vi "Create_TreeNode_PN.vi"(1 "Input cluster":T1) -> (0 "TreeNode out":T2)   [LabVIEW 2011]
uses:
  TreeNode2D.ctl
  TreeNode2D Input Cluster.ctl
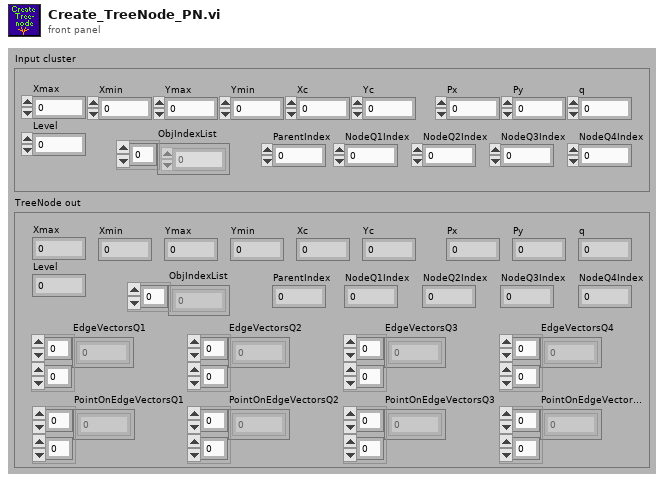
[diagram p1: front panel]
types:
  T1 = typedef "TreeNode2D Input Cluster.ctl" = cluster{"Xmax":dbl, "Xmin":dbl, "Ymax":dbl, "Ymin":dbl, "Xc":dbl, "Yc":dbl, "Px":dbl, "Py":dbl, "q":dbl, "Level":i32, "ObjIndexList":i32[], "ParentIndex":i32, "NodeQ1Index":i32, "NodeQ2Index":i32, "NodeQ3Index":i32, "NodeQ4Index":i32}
  T2 = typedef "TreeNode2D.ctl" = cluster{"Xmax":dbl, "Xmin":dbl, "Ymax":dbl, "Ymin":dbl, "Xc":dbl, "Yc":dbl, "Px":dbl, "Py":dbl, "q":dbl, "Level":i32, "ObjIndexList":i32[], "ParentIndex":i32, "NodeQ1Index":i32, "NodeQ2Index":i32, "NodeQ3Index":i32, "NodeQ4Index":i32, "EdgeVectorsQ1":dbl[][], "EdgeVectorsQ2":dbl[][], "EdgeVectorsQ3":dbl[][], "EdgeVectorsQ4":dbl[][], "PointOnEdgeVectorsQ1":dbl[][], "PointOnEdgeVectorsQ2":dbl[][], "PointOnEdgeVectorsQ3":dbl[][], "PointOnEdgeVectorsQ4":dbl[][]}
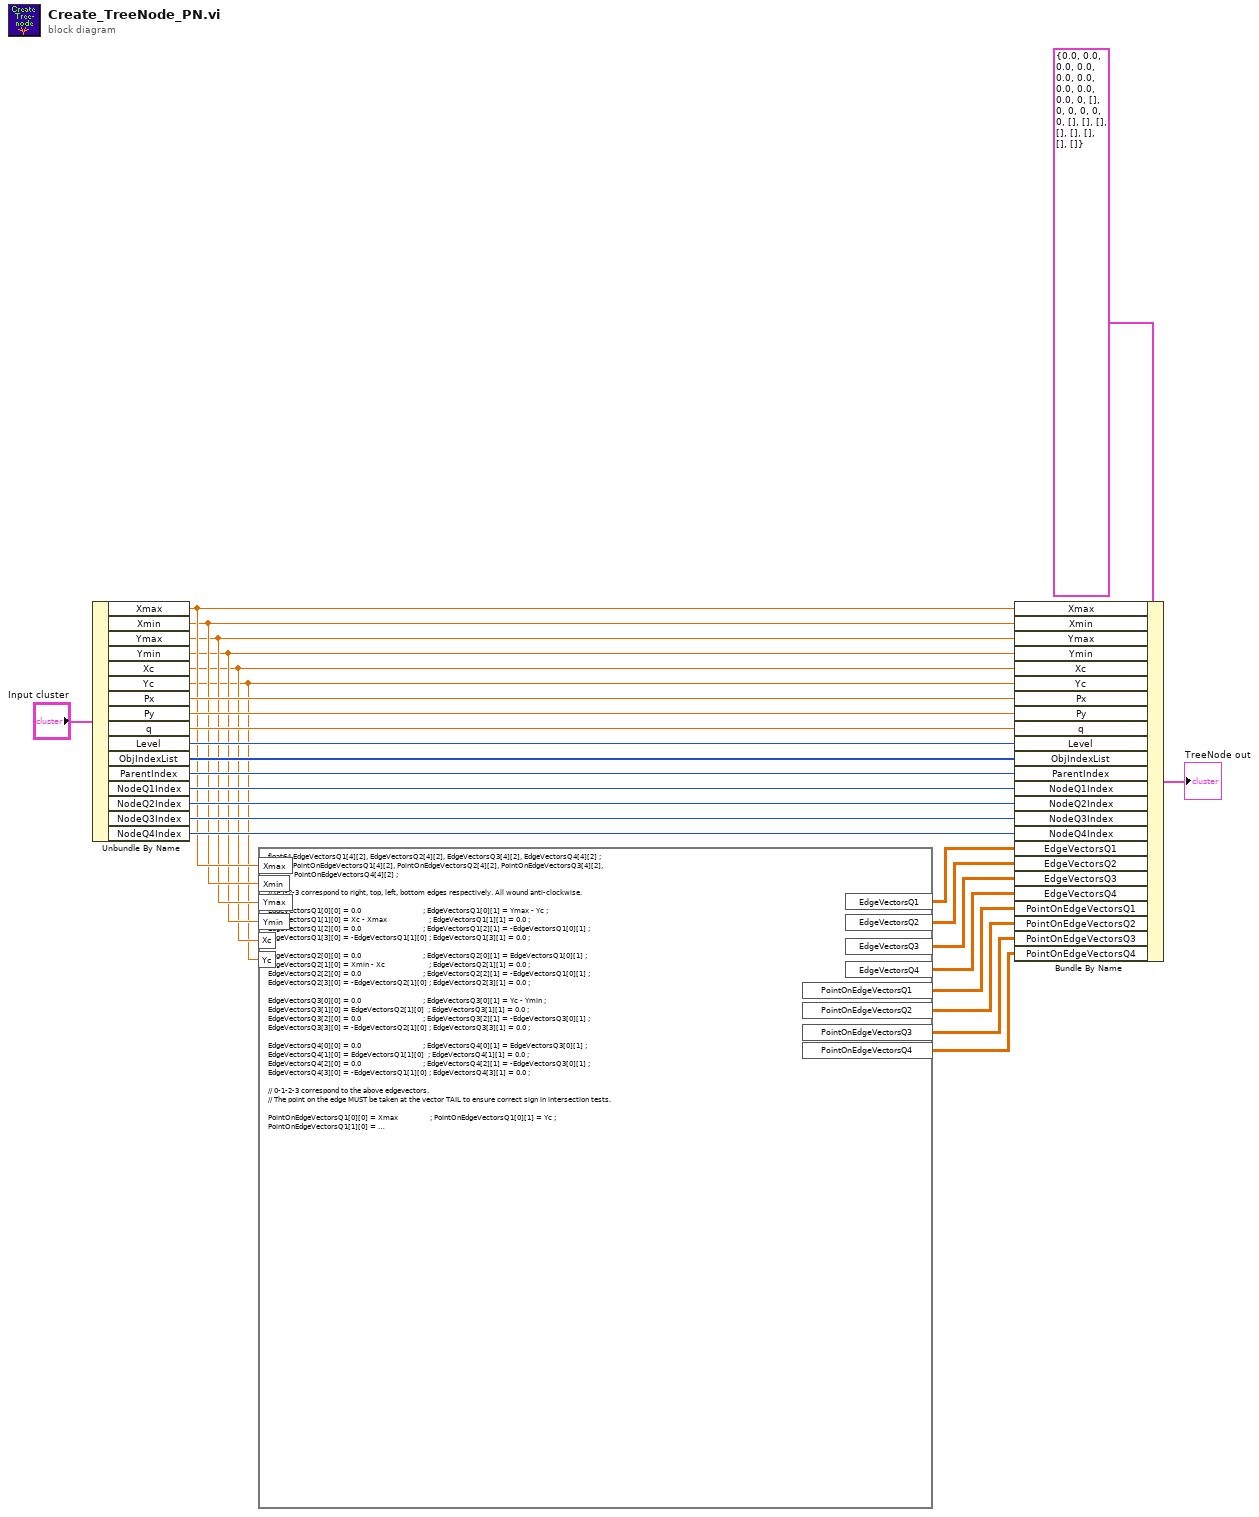
[diagram p0: block diagram]
diagram:
  n1 = Unbundle By Name("Input cluster") -> ("Xmax"=w13:dbl, "Xmin"=w12:dbl, "Ymax"=w11:dbl, "Ymin"=w10:dbl, "Xc"=w9:dbl, "Yc"=w8:dbl, "Px"=w24:dbl, "Py"=w23:dbl, "q"=w22:dbl, "Level"=w21:i32, "ObjIndexList"=w20:i32[], "ParentIndex"=w19:i32, "NodeQ1Index"=w18:i32, "NodeQ2Index"=w17:i32, "NodeQ3Index"=w16:i32, "NodeQ4Index"=w15:i32)
  n2 = formula code="float64 EdgeVectorsQ1[4][2], EdgeVectorsQ2[4][2], EdgeVectorsQ3[4][2], EdgeVectorsQ4[4][2] ;\nfloat64 PointOnEdgeVectorsQ1[4][2], PointOnEdgeVectorsQ2[4][2], PointOnEdgeVectorsQ3[4][2], \n             PointOnEdgeVectorsQ4[4][2] ;\n\n// 0-1-2-3 correspond to right, top, left, bottom edges respectively. All wound anti-clockwise.\n\nEdgeVectorsQ1[0][0] = 0.0                               ; EdgeVectorsQ1[0][1] = Ymax - Yc ;\nEdgeVectorsQ1[1][0] = Xc - Xmax                     ; EdgeVectorsQ1[1][1] = 0.0 ;\nEdgeVectorsQ1[2][0] = 0.0                               ; EdgeVectorsQ1[2][1] = -EdgeVectorsQ1[0][1] ;\nEdgeVectorsQ1[3][0] = -EdgeVectorsQ1[1][0] ; EdgeVectorsQ1[3][1] = 0.0 ;\n\nEdgeVectorsQ2[0][0] = 0.0                               ; EdgeVectorsQ2[0][1] = EdgeVectorsQ1[0][1] ;\nEdgeVectorsQ2[1][0] = Xmin - Xc                      ; EdgeVectorsQ2[1][1] = 0.0 ;\nEdgeVectorsQ2[2][0] = 0.0                               ; EdgeVectorsQ2[2][1] = -EdgeVectorsQ1[0][1] ;\nEdgeVectorsQ2[3][0] = -EdgeVectorsQ2[1][0] ; EdgeVectorsQ2[3][1] = 0.0 ;\n\nEdgeVectorsQ3[0][0] = 0.0                               ; EdgeVectorsQ3[0][1] = Yc - Ymin ;\nEdgeVectorsQ3[1][0] = EdgeVectorsQ2[1][0]  ; EdgeVectorsQ3[1][1] = 0.0 ;\nEdgeVectorsQ3[2][0] = 0.0                               ; EdgeVectorsQ3[2][1] = -EdgeVectorsQ3[0][1] ;\nEdgeVectorsQ3[3][0] = -EdgeVectorsQ2[1][0] ; EdgeVectorsQ3[3][1] = 0.0 ;\n\nEdgeVectorsQ4[0][0] = 0.0                               ; EdgeVectorsQ4[0][1] = EdgeVectorsQ3[0][1] ;\nEdgeVectorsQ4[1][0] = EdgeVectorsQ1[1][0]  ; EdgeVectorsQ4[1][1] = 0.0 ;\nEdgeVectorsQ4[2][0] = 0.0                               ; EdgeVectorsQ4[2][1] = -EdgeVectorsQ3[0][1] ;\nEdgeVectorsQ4[3][0] = -EdgeVectorsQ1[1][0] ; EdgeVectorsQ4[3][1] = 0.0 ;\n\n// 0-1-2-3 correspond to the above edgevectors.\n// The point on the edge MUST be taken at the vector TAIL to ensure correct sign in intersection tests.\n\nPointOnEdgeVectorsQ1[0][0] = Xmax                ; PointOnEdgeVectorsQ1[0][1] = Yc ;\nPointOnEdgeVectorsQ1[1][0] = Xmax                ; PointOnEdgeVectorsQ1[1][1] = Ymax ;\nPointOnEdgeVectorsQ1[2][0] = Xc                     ; PointOnEdgeVectorsQ1[2][1] = Ymax ;\nPointOnEdgeVectorsQ1[3][0] = Xc                     ; PointOnEdgeVectorsQ1[3][1] = Yc ;\n\nPointOnEdgeVectorsQ2[0][0] = Xc                     ; PointOnEdgeVectorsQ2[0][1] = Yc ;\nPointOnEdgeVectorsQ2[1][0] = Xc                     ; PointOnEdgeVectorsQ2[1][1] = Ymax ;\nPointOnEdgeVectorsQ2[2][0] = Xmin                 ; PointOnEdgeVectorsQ2[2][1] = Ymax ;\nPointOnEdgeVectorsQ2[3][0] = Xmin                 ; PointOnEdgeVectorsQ2[3][1] = Yc ;\n\nPointOnEdgeVectorsQ3[0][0] = Xc                     ; PointOnEdgeVectorsQ3[0][1] = Ymin ;\nPointOnEdgeVectorsQ3[1][0] = Xc                     ; PointOnEdgeVectorsQ3[1][1] = Yc ;\nPointOnEdgeVectorsQ3[2][0] = Xmin                 ; PointOnEdgeVectorsQ3[2][1] = Yc ;\nPointOnEdgeVectorsQ3[3][0] = Xmin                 ; PointOnEdgeVectorsQ3[3][1] = Ymin ;\n\nPointOnEdgeVectorsQ4[0][0] = Xmax                ; PointOnEdgeVectorsQ4[0][1] = Ymin ;\nPointOnEdgeVectorsQ4[1][0] = Xmax                ; PointOnEdgeVectorsQ4[1][1] = Yc ;\nPointOnEdgeVectorsQ4[2][0] = Xc                     ; PointOnEdgeVectorsQ4[2][1] = Yc ;\nPointOnEdgeVectorsQ4[3][0] = Xc                     ; PointOnEdgeVectorsQ4[3][1] = Ymin ;"("Xmax"=w13, "Xmin"=w12, "Ymax"=w11, "Ymin"=w10, "Xc"=w9, "Yc"=w8) -> ("EdgeVectorsQ1"=w14:dbl[][], "EdgeVectorsQ2"=w7:dbl[][], "EdgeVectorsQ3"=w6:dbl[][], "EdgeVectorsQ4"=w5:dbl[][], "PointOnEdgeVectorsQ1"=w4:dbl[][], "PointOnEdgeVectorsQ2"=w3:dbl[][], "PointOnEdgeVectorsQ3"=w2:dbl[][], "PointOnEdgeVectorsQ4"=w1:dbl[][])
  n3 = Bundle By Name(cluster=T2 {"Xmax"=0.0, "Xmin"=0.0, "Ymax"=0.0, "Ymin"=0.0, "Xc"=0.0, "Yc"=0.0, "Px"=0.0, "Py"=0.0, "q"=0.0, "Level"=0, "ObjIndexList"=[], "ParentIndex"=0, "NodeQ1Index"=0, "NodeQ2Index"=0, "NodeQ3Index"=0, "NodeQ4Index"=0, "EdgeVectorsQ1"=[], "EdgeVectorsQ2"=[], "EdgeVectorsQ3"=[], "EdgeVectorsQ4"=[], "PointOnEdgeVectorsQ1"=[], "PointOnEdgeVectorsQ2"=[], "PointOnEdgeVectorsQ3"=[], "PointOnEdgeVectorsQ4"=[]} ("TreeNode out"), "Xmax"=w13, "Xmin"=w12, "Ymax"=w11, "Ymin"=w10, "Xc"=w9, "Yc"=w8, "Px"=w24, "Py"=w23, "q"=w22, "Level"=w21, "ObjIndexList"=w20, "ParentIndex"=w19, "NodeQ1Index"=w18, "NodeQ2Index"=w17, "NodeQ3Index"=w16, "NodeQ4Index"=w15, "EdgeVectorsQ1"=w14, "EdgeVectorsQ2"=w7, "EdgeVectorsQ3"=w6, "EdgeVectorsQ4"=w5, "PointOnEdgeVectorsQ1"=w4, "PointOnEdgeVectorsQ2"=w3, "PointOnEdgeVectorsQ3"=w2, "PointOnEdgeVectorsQ4"=w1) -> (→"TreeNode out":T2)
